vi "GetXL_CellValue_Dbl.vi"(8 "error in":errorcluster, 9 "End":cluster{"Column":i32, "Row":i32}, 10 "Start":cluster{"Column":i32, "Row":i32}, 11 "Refnum Cluster In":T1) -> (0 "error out":errorcluster, 2 "data":dbl, 3 "Refnum Cluster Out":T1)   [LabVIEW 2017, in "excel_configuration.lvlib"]
uses:
  excel_configuration.lvlib
  bfe4c074-56a8-4928-803a-ddef92461171.vi
  <vilib>/Utility/error.llb/Clear Errors.vi
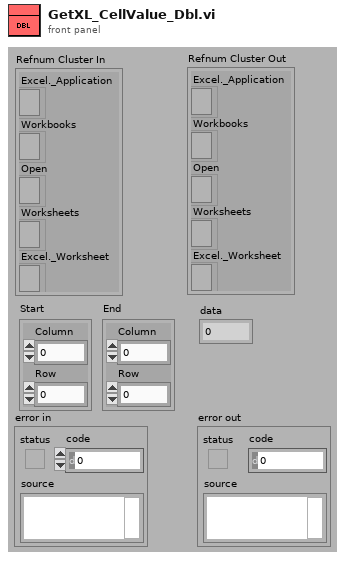
[diagram p1: front panel]
types:
  T1 = cluster{"Excel._Application":refnum<k7>, "Workbooks":refnum<k7>, "Open":refnum<k7>, "Worksheets":refnum<k7>, "Excel._Worksheet":refnum<k7>}
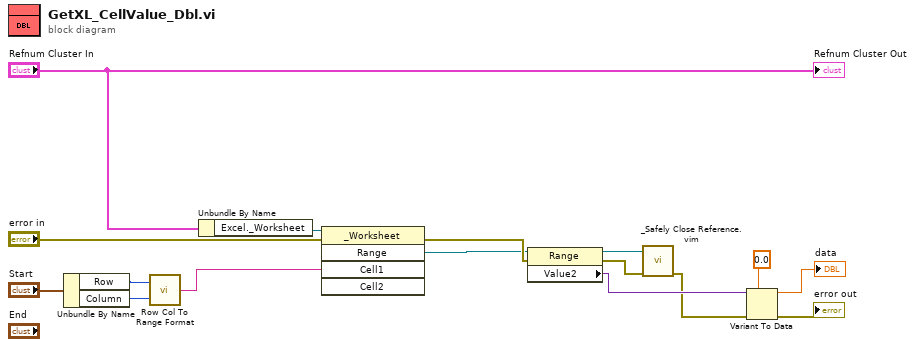
[diagram p0: block diagram]
diagram:
  n1 = Unbundle By Name("Start") -> ("Row"=w10:i32, "Column"=w9:i32)
  n2 = call "Row Col To Range Format.vi"("Column"=w9, "Row"=w10) -> ("Output String"=w8:string)
  n3 = Unbundle By Name("Refnum Cluster In") -> ("Excel._Worksheet"=w2:refnum<k7>)
  n4 = invoke class="_Worksheet" method="Range"(reference=w2, error in="error in", "Cell1"=w8) -> (error out=w15:errorcluster, "Range"=w14:refnum<k7>)  [unwired: 2 in, 3 out]
  n5 = property class="Range"(reference=w14, error in=w15) -> (reference out=w13:refnum<k7>, error out=w12:errorcluster, "Value2"=w7:variant)
  n6 = call "_Safely Close Reference.vim"("error in (no error)"=w12, "Automation Refnum in"=w13) -> ("error out"=w6:errorcluster)  [unwired: 9 in]
  n7 = Variant To Data(error in=w6, type=0.0, Variant=w7) -> (data=→"data":dbl, error out=→"error out":errorcluster)
  "Refnum Cluster Out" <- "Refnum Cluster In"
